vi "DynamicEventRegister.vi"() -> ()   [LabVIEW 2014]
panel:
  in  "Text Ring":u16(ring) items=["None", "FormA", "FormB"]
  out "Time":u32
  in  "ButtonB":bool
  in  "ButtonA":bool
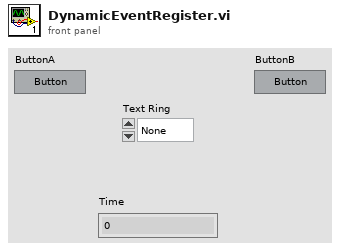
[diagram p1: front panel]
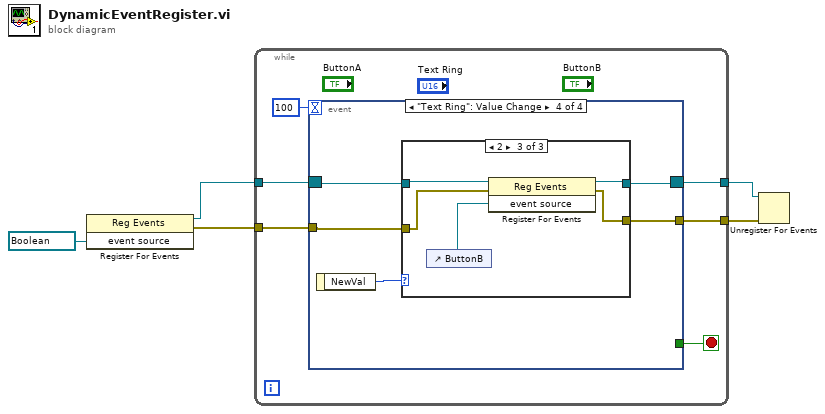
[diagram p0: block diagram]
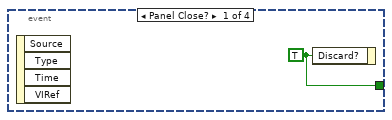
[diagram p2: hidden frame]
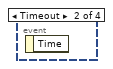
[diagram p3: hidden frame]
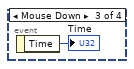
[diagram p4: hidden frame]
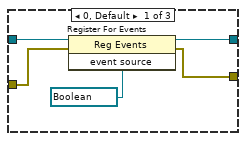
[diagram p5: hidden frame]
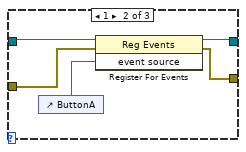
[diagram p6: hidden frame]
diagram:
  n1 = register-events(refnum<vi> refnum ("event source")) -> (reference out=w4:refnum<event-registration>, error out=w5:errorcluster)  [unwired: 2 in]
  n2 = while {
    tunnel: w5 -> [w9]
    tunnel: w4 -> [w8]
    tunnel: [w7] -> w2
    tunnel: [w6] -> w1
    stop <- w10 stop-if-true
    n3 = event shown="[3] \"Text Ring\": Value Change" {
      selector: w8 -> [_ _ _ w16]
      dyn-events: [_ _ _ w17] -> w6
      timeout: 100 -> [_ _ _ _]
      tunnel: [w12 _ _ _] -> w10
      tunnel: w9 -> [_ _ _ w15]
      tunnel: [_ _ _ w14] -> w7
      event Panel Close? {
        w12 = TRUE ("Discard?")
        n4 = event-data() -> ()  [unwired: 1 in, 4 out]
        n5 = event-data("Discard?"=w12) -> ()  [unwired: 1 in, 1 out]
      }
      event Timeout {
        n6 = event-data() -> ()  [unwired: 1 in, 1 out]
      }
      event Mouse Down {
        n7 = event-data() -> ("Time"=→"Time":u32)  [unwired: 1 in]
      }
      event "Text Ring": Value Change {
        n8 = event-data() -> ("NewVal"=w18:u16)  [unwired: 1 in]
        n9 = case shown="2" w18 {
          tunnel: [w22 w27 w32] -> w17
          tunnel: w16 -> [w23 w28 w33]
          tunnel: w15 -> [w20 w25 w30]
          tunnel: [w19 w24 w29] -> w14
          frame 0, Default {
            n10 = register-events(reference=w23, error in=w20, refnum<vi> refnum ("event source")) -> (reference out=w22:refnum<event-registration>, error out=w19:errorcluster)
          }
          frame 1 {
            n11 = control-ref of="ButtonA"() -> (w26:refnum<vi>)
            n12 = register-events(reference=w28, error in=w25, w26) -> (reference out=w27:refnum<event-registration>, error out=w24:errorcluster)
          }
          frame 2 {
            n13 = control-ref of="ButtonB"() -> (w31:refnum<vi>)
            n14 = register-events(reference=w33, error in=w30, w31) -> (reference out=w32:refnum<event-registration>, error out=w29:errorcluster)
          }
        }
      }
    }
  }
  n15 = Unregister For Events(event registration refnum=w1, error in=w2) -> ()  [unwired: 1 out]
